vi "Read Global Locked.vi"(7 "Semaphore Timeout":i32=-1, 8 "error in (no error)":errorcluster, 11 "DriveMotorsRight in":refnum<class "DriveMotorsRight.lvclass">) -> (0 "error out":errorcluster, 1 "Semaphore Timed Out":bool, 2 "Global":refnum<class "System.lvclass">, 3 "DriveMotorsRight out":refnum<class "DriveMotorsRight.lvclass">)   [LabVIEW 2013]
uses:
  Robot Global Data.vi
  System/System.lvclass
  DriveMotorsRight.lvclass
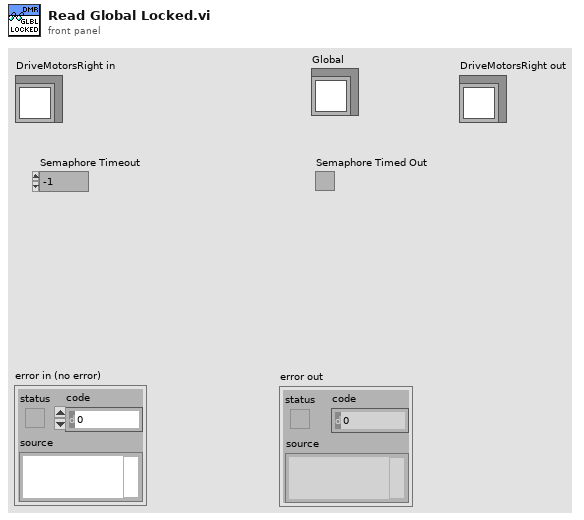
[diagram p1: front panel]
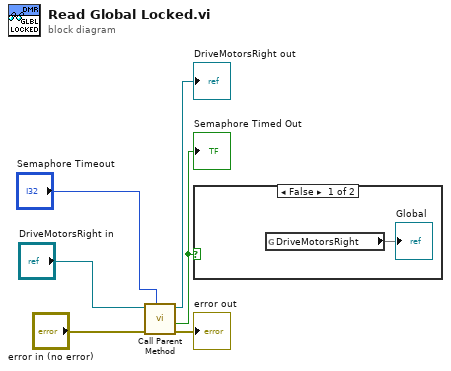
[diagram p0: block diagram]
diagram:
  n1 = call-parent "Call Parent Method"("Semaphore Timeout"="Semaphore Timeout", "error in (no error)"="error in (no error)", "System in"="DriveMotorsRight in") -> ("error out"=→"error out":errorcluster, "Semaphore Timed Out"=w1:bool, "System out"=→"DriveMotorsRight out":refnum<class "DriveMotorsRight.lvclass">)  [unwired: 5 in, 1 out]
  "Semaphore Timed Out" <- w1
  n2 = case shown="False" w1 {
    frame False {
      n3 = global read "Robot Global Data.vi" "DriveMotorsRight"() -> (→"Global")
    }
    frame True {
    }
  }
